vi "Open_GDS_Help.vi"   [LabVIEW 2020]
doc: "GOOP Help"
uses:
  <vilib>/Platform/browser.llb/Open URL in Default Browser (path).vi
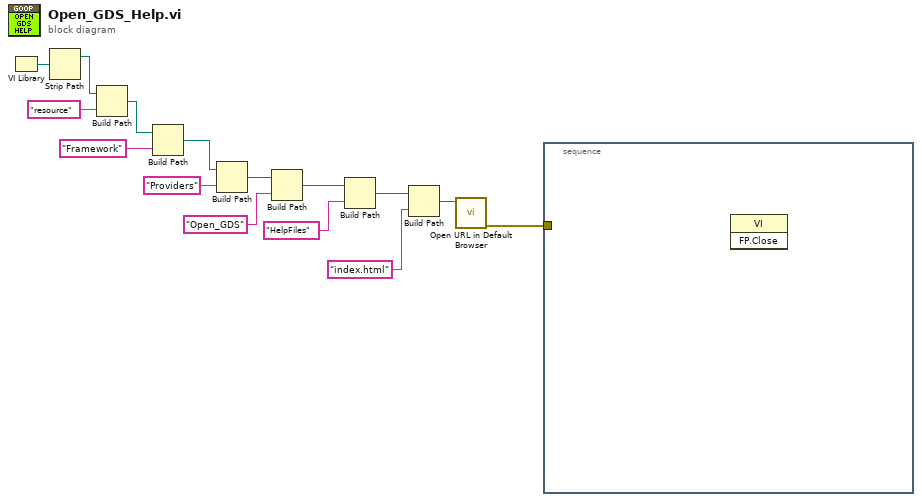
[diagram p0: block diagram]
diagram:
  n1 = VI Library() -> (path=w6:path)
  n2 = Strip Path(path=w6) -> (stripped path=w13:path)  [unwired: 1 out]
  n3 = Build Path(base path=w13, name or relative path="resource") -> (appended path=w7:path)
  n4 = Build Path(base path=w7, name or relative path="Framework") -> (appended path=w8:path)
  n5 = Build Path(base path=w8, name or relative path="Providers") -> (appended path=w15:path)
  n6 = Build Path(base path=w15, name or relative path="Open_GDS") -> (appended path=w14:path)
  n7 = Build Path(base path=w14, name or relative path="HelpFiles") -> (appended path=w4:path)
  n8 = Build Path(base path=w4, name or relative path="index.html") -> (appended path=w3:path)
  n9 = call-poly <vilib>:"Open URL in Default Browser.vi"("path"=w3) -> ("error out"=w1:errorcluster)  [unwired: 5 in, 1 out]
  n10 = stacked-sequence {
    tunnel: w1 -> [_]
    frame #0 {
      n11 = invoke class="VI" method="FP.Close"() -> ()  [unwired: 3 in, 3 out]
    }
  }
